vi "Generate Event.vi"(4 "Error In":errorcluster, 7 "event data":T1) -> (0 "Error Out":errorcluster)   [LabVIEW 2014, in "Pass Data.lvlib"]
uses:
  Pass Data.lvlib
  Event Data.ctl
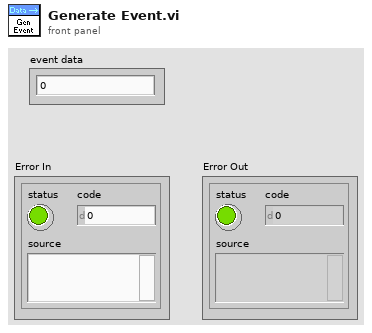
[diagram p1: front panel]
types:
  T1 = typedef "Pass Data.lvlib/Event Data.ctl" = dbl
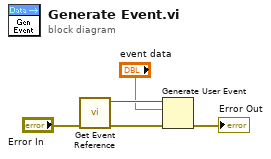
[diagram p0: block diagram]
diagram:
  n1 = call "Get Event Reference.vi"("error in (no error)"="Error In") -> ("error out"=w4:errorcluster, "Pass Data"=w3:refnum<user-event>)  [unwired: 5 in]
  n2 = Generate User Event(user event=w3, event data cluster="event data", error in=w4) -> (error out=→"Error Out":errorcluster)  [unwired: 1 in, 1 out]
